vi "dll.midi_file_get_event.vi"(8 "error in (no error)":errorcluster, 9 "Event Index":i32, 10 "Track Index":i32, 11 "midi file in":refnum<class "midi file.lvclass">) -> (0 "error out":errorcluster, 2 "Event Details":T1, 3 "midi file out":refnum<class "midi file.lvclass">)   [LabVIEW 2020, in "midi file.lvclass"]
uses:
  midi file.lvclass
  event info.ctl
  event type.ctl
  midi file.lvclass/midi file.ctl
  shared/midi shared.lvlib
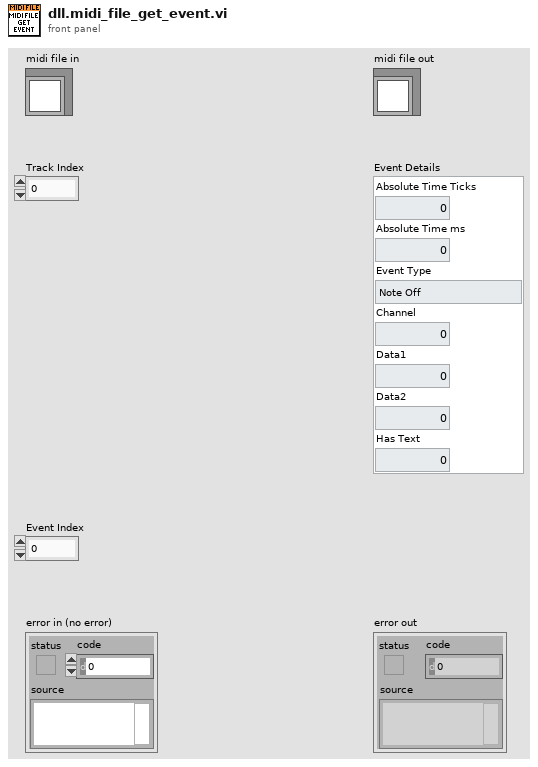
[diagram p1: front panel]
types:
  T1 = typedef "midi file.lvclass/event info.ctl" = cluster{"Absolute Time Ticks":u32, "Absolute Time ms":dbl, "Event Type":T2, "Channel":u8, "Data1":u8, "Data2":u8, "Has Text":i32}
  T2 = typedef "midi file.lvclass/event type.ctl" = enum32{"Note Off", "Note On", "Polyphonic Aftertouch", "Control Change", "Program Change", "Channel Aftertouch", "Pitch Bend", "System Exclusive", "8 - undefined", "9 - undefined", "10 - undefined", "11 - undefined", "12 - undefined", "13 - undefined", "14 - undefined", "15 - undefined", "16 - undefined", "17 - undefined", "18 - undefined", "19 - undefined", "20 - undefined", "21 - undefined", "22 - undefined", "23 - undefined", "24 - undefined", "25 - undefined", "26 - undefined", "27 - undefined", "28 - undefined", "29 - undefined", "30 - undefined", "31 - undefined", "32 - undefined", "33 - undefined", "34 - undefined", "35 - undefined", "36 - undefined", "37 - undefined", "38 - undefined", "39 - undefined", "40 - undefined", "41 - undefined", "42 - undefined", "43 - undefined", "44 - undefined", "45 - undefined", "46 - undefined", "47 - undefined", "48 - undefined", "49 - undefined", "50 - undefined", "51 - undefined", "52 - undefined", "53 - undefined", "54 - undefined", "55 - undefined", "56 - undefined", "57 - undefined", "58 - undefined", "59 - undefined", "60 - undefined", "61 - undefined", "62 - undefined", "63 - undefined", "64 - undefined", "65 - undefined", "66 - undefined", "67 - undefined", "68 - undefined", "69 - undefined", "70 - undefined", "71 - undefined", "72 - undefined", "73 - undefined", "74 - undefined", "75 - undefined", "76 - undefined", "77 - undefined", "78 - undefined", "79 - undefined", "80 - undefined", "81 - undefined", "82 - undefined", "83 - undefined", "84 - undefined", "85 - undefined", "86 - undefined", "87 - undefined", "88 - undefined", "89 - undefined", "90 - undefined", "91 - undefined", "92 - undefined", "93 - undefined", "94 - undefined", "95 - undefined", "96 - undefined", "97 - undefined", "98 - undefined", "99 - undefined", "Meta: Sequence Number", "Meta: Text", "Meta: Copyright", "Meta: Track Name", "Meta: Instrument Name", "Meta: Lyric", "Meta: Marker", "Meta: Cue Point", "Meta: Channel Prefix", "Meta: End of Track", "Meta: Set Tempo", "Meta: SMPTE Offset", "Meta: Time Signature", "Meta: Key Signature", "Meta: Sequencer Specific", "115 - undefined", "116 - undefined", "117 - undefined", "118 - undefined", "119 - undefined", "120 - undefined", "121 - undefined", "122 - undefined", "123 - undefined", "124 - undefined", "125 - undefined", "126 - undefined", "127 - undefined", "128 - undefined", "129 - undefined", "130 - undefined", "131 - undefined", "132 - undefined", "133 - undefined", "134 - undefined", "135 - undefined", "136 - undefined", "137 - undefined", "138 - undefined", "139 - undefined", "140 - undefined", "141 - undefined", "142 - undefined", "143 - undefined", "144 - undefined", "145 - undefined", "146 - undefined", "147 - undefined", "148 - undefined", "149 - undefined", "150 - undefined", "151 - undefined", "152 - undefined", "153 - undefined", "154 - undefined", "155 - undefined", "156 - undefined", "157 - undefined", "158 - undefined", "159 - undefined", "160 - undefined", "161 - undefined", "162 - undefined", "163 - undefined", "164 - undefined", "165 - undefined", "166 - undefined", "167 - undefined", "168 - undefined", "169 - undefined", "170 - undefined", "171 - undefined", "172 - undefined", "173 - undefined", "174 - undefined", "175 - undefined", "176 - undefined", "177 - undefined", "178 - undefined", "179 - undefined", "180 - undefined", "181 - undefined", "182 - undefined", "183 - undefined", "184 - undefined", "185 - undefined", "186 - undefined", "187 - undefined", "188 - undefined", "189 - undefined", "190 - undefined", "191 - undefined", "192 - undefined", "193 - undefined", "194 - undefined", "195 - undefined", "196 - undefined", "197 - undefined", "198 - undefined", "199 - undefined", "200 - undefined", "201 - undefined", "202 - undefined", "203 - undefined", "204 - undefined", "205 - undefined", "206 - undefined", "207 - undefined", "208 - undefined", "209 - undefined", "210 - undefined", "211 - undefined", "212 - undefined", "213 - undefined", "214 - undefined", "215 - undefined", "216 - undefined", "217 - undefined", "218 - undefined", "219 - undefined", "220 - undefined", "221 - undefined", "222 - undefined", "223 - undefined", "224 - undefined", "225 - undefined", "226 - undefined", "227 - undefined", "228 - undefined", "229 - undefined", "230 - undefined", "231 - undefined", "232 - undefined", "233 - undefined", "234 - undefined", "235 - undefined", "236 - undefined", "237 - undefined", "238 - undefined", "239 - undefined", "240 - undefined", "241 - undefined", "242 - undefined", "243 - undefined", "244 - undefined", "245 - undefined", "246 - undefined", "247 - undefined", "248 - undefined", "249 - undefined", "250 - undefined", "251 - undefined", "252 - undefined", "253 - undefined", "254 - undefined", "Unknown"}
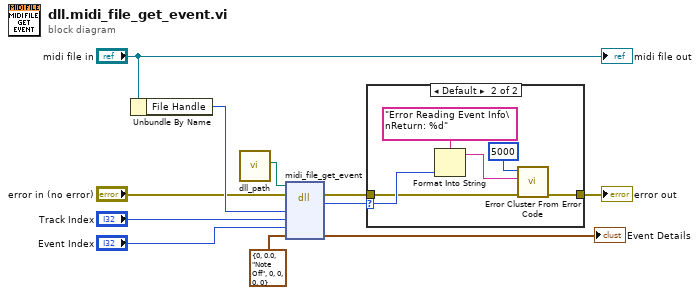
[diagram p0: block diagram]
diagram:
  n1 = Unbundle By Name("midi file in") -> ("File Handle"=w7:i32)
  n2 = call "dll_path.vi"() -> ("dll"=w11:path)  [unwired: 11 in]
  n3 = dll-call lib="C:/code/LabVIEW-MIDI-XPLAT/dist/TomMIDIllan_*.*" fn="midi_file_get_event"(path in=w11, error in="error in (no error)", "File Handle"=w7, "Track Index"="Track Index", "Event Index"="Event Index", "Event Cluster"=T1 {"Absolute Time Ticks"=0, "Absolute Time ms"=0.0, "Event Type"=enum."Note Off", "Channel"=0, "Data1"=0, "Data2"=0, "Has Text"=0} ("Event Info")) -> (error out=w10:errorcluster, "Error code"=w9:i32, "Event Cluster"=→"Event Details":T1)  [unwired: 4 in, 1 out]
  n4 = case shown="Default" w9 {
    selector: w9 -> [_ w15]
    tunnel: w10 -> [w12 w14]
    tunnel: [w12 w13] -> w5
    frame 0.. {
    }
    frame Default {
      n5 = Format Into String(format string="Error Reading Event Info\nReturn: %d", w15) -> (resulting string=w16:string)  [unwired: 2 in, 1 out]
      n6 = call <vilib>:"Error Cluster From Error Code.vi"("error in (no error)"=w14, "error message (\"\")"=w16, "error code (0)"=5000) -> ("error out"=w13:errorcluster)  [unwired: 6 in]
    }
  }
  "error out" <- w5
  "midi file out" <- "midi file in"
